vi "Start Shooter Implementation.vi"(8 "Deadband (RPM)":dbl, 10 "Shooter Velocity Setpoint In":dbl, 11 "Shooter":T1) -> (0 "Finished?":bool, 3 "Shooter Velocity Setpoint Out":dbl)   [LabVIEW 2019]
uses:
  <vilib>/Rock Robotics/WPI/MotorControl/WPI_MotorControlDeviceRef.ctl
  <vilib>/Rock Robotics/WPI/MotorControl/WPI_MotorControlType.ctl
  <vilib>/Rock Robotics/SystemInterfaces/DIO/FPGA_DIOPWMChannel.ctl
  <vilib>/Rock Robotics/WPI/PWM/WPI_PWMDeadband.ctl
  <vilib>/Rock Robotics/SystemInterfaces/DIO/FPGA_DIOChannel.ctl
  Turret Published Globals.vi
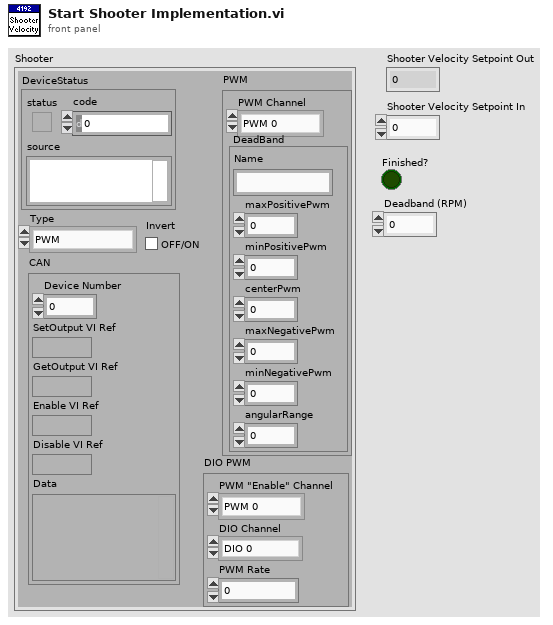
[diagram p1: front panel]
types:
  T1 = typedef "WPI_MotorControlDeviceRef.ctl" = cluster{"DeviceStatus":errorcluster, "Type":T2, "PWM":cluster{"PWM Channel":T3, "DeadBand":T4}, "CAN":cluster{"Device Number":u8, "SetOutput VI Ref":variant, "GetOutput VI Ref":variant, "Enable VI Ref":variant, "Disable VI Ref":variant, "Data":variant}, "Invert":bool, "DIO PWM":cluster{"PWM \"Enable\" Channel":T3, "DIOChannel":T5, "PWM Rate":dbl}}
  T2 = typedef "WPI_MotorControlType.ctl" = enum16{"PWM", "CAN", "DIO PWM"}
  T3 = typedef "FPGA_DIOPWMChannel.ctl" = enum8{"PWM 0", "PWM 1", "PWM 2", "PWM 3", "PWM 4", "PWM 5", "PWM 6", "PWM 7", "PWM 8", "PWM 9", "PWM MXP 0", "PWM MXP 1", "PWM MXP 2", "PWM MXP 3", "PWM MXP 4", "PWM MXP 5", "PWM MXP 6", "PWM MXP 7", "PWM MXP 8", "PWM MXP 9", "Invalid"}
  T4 = typedef "WPI_PWMDeadband.ctl" = cluster{"Name":string, "maxPositivePwm":i32, "minPositivePwm":i32, "centerPwm":i32, "maxNegativePwm":i32, "minNegativePwm":i32, "angularRange":u16}
  T5 = typedef "FPGA_DIOChannel.ctl" = enum8{"DIO 0", "DIO 1", "DIO 2", "DIO 3", "DIO 4", "DIO 5", "DIO 6", "DIO 7", "DIO 8", "DIO 9", "DIO MXP 0", "DIO MXP 1", "DIO MXP 2", "DIO MXP 3", "DIO MXP 4", "DIO MXP 5", "DIO MXP 6", "DIO MXP 7", "DIO MXP 8", "DIO MXP 9", "DIO MXP 10", "DIO MXP 11", "DIO MXP 12", "DIO MXP 13", "DIO MXP 14", "DIO MXP 15", "SPI Port CS1", "SPI Port CS2", "SPI Port CS3", "SPI Port MISO", "SPI Port MOSI", "Invalid"}
  T6 = cluster{"Sensor Velocity":dbl, "Setpoint":dbl, "Applied Output":dbl}
  T7 = cluster{"Shooter Velocity":cluster{"Sensor Velocity":dbl, "Setpoint":dbl, "Applied Output":dbl}, "Turret Position":cluster{"output":dbl, "Horizontal Offset":dbl}, "Hood Position":cluster{"Sensor Velocity":dbl, "Setpoint":dbl, "Applied Output":dbl}, "Shooter PID Constants":cluster{"P Gain":dbl, "I Gain":dbl, "D Gain":dbl, "F Gain":dbl, "I Zone":dbl, "Min Output":dbl, "Max Output":dbl}, "Hood PID Constants":cluster{"P Gain":dbl, "I Gain":dbl, "D Gain":dbl, "F Gain":dbl, "I Zone":dbl, "Min Output":dbl, "Max Output":dbl}, "Turret PID Constants":cluster{"P Gain":dbl, "I Gain":dbl, "D Gain":dbl, "F Gain":dbl, "I Zone":dbl, "Min Output":dbl, "Max Output":dbl}, "Limelight PID Gains":cluster{"proportional gain (Kc)":dbl, "integral time (Ti, min)":dbl, "derivative time (Td, min)":dbl}}
  T8 = cluster{"Shooter Up To Speed?":bool, "Aligned With Target?":bool, "Hood at Angle?":bool, "Shooting?":bool, "Hood Angle":dbl, "Turret Angle":dbl}
  T9 = cluster{"P Gain":dbl, "I Gain":dbl, "D Gain":dbl, "F Gain":dbl, "I Zone":dbl, "Min Output":dbl, "Max Output":dbl}
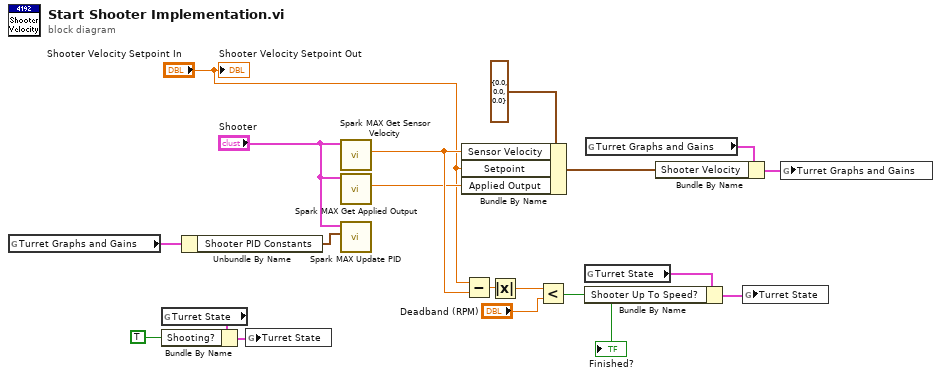
[diagram p0: block diagram]
diagram:
  n1 = global read "Turret Published Globals.vi" "Turret Graphs and Gains"() -> (w11:T7)
  n2 = global read "Turret Published Globals.vi" "Turret State"() -> (w14:T8)
  n3 = Bundle By Name(cluster=w14, "Shooting?"=TRUE) -> (w13:T8)
  n4 = Unbundle By Name(w11) -> ("Shooter PID Constants"=w10:T9)
  n5 = global write "Turret Published Globals.vi" "Turret State"(w13) -> ()
  n6 = call <vilib>:"Spark MAX Get Sensor Velocity.vi"("MotorControlDevRef in"="Shooter") -> ("Sensor Velocity"=w17:dbl)  [unwired: 7 in, 3 out]
  n7 = call <vilib>:"Spark MAX Get Applied Output.vi"("MotorControlDevRef in"="Shooter") -> ("Applied Output"=w16:dbl)  [unwired: 7 in, 3 out]
  n8 = call "Spark MAX Update PID.vi"("MotorControlDeviceRef"="Shooter", "PID Constants"=w10) -> ()  [unwired: 8 in]
  n9 = Bundle By Name(cluster=T6 {"Sensor Velocity"=0.0, "Setpoint"=0.0, "Applied Output"=0.0} ("Shooter Velocity"), "Sensor Velocity"=w17, "Setpoint"="Shooter Velocity Setpoint In", "Applied Output"=w16) -> (w7:T6)
  n10 = Subtract(x="Shooter Velocity Setpoint In", y=w17) -> (x-y=w18:dbl)
  n11 = Absolute Value(x=w18) -> (abs(x)=w19:dbl)
  n12 = Less?(x=w19, y="Deadband (RPM)") -> (x < y?=w3:bool)
  "Finished?" <- w3
  n13 = global read "Turret Published Globals.vi" "Turret State"() -> (w4:T8)
  n14 = Bundle By Name(cluster=w4, "Shooter Up To Speed?"=w3) -> (w5:T8)
  n15 = global read "Turret Published Globals.vi" "Turret Graphs and Gains"() -> (w8:T7)
  n16 = Bundle By Name(cluster=w8, "Shooter Velocity"=w7) -> (w9:T7)
  n17 = global write "Turret Published Globals.vi" "Turret State"(w5) -> ()
  n18 = global write "Turret Published Globals.vi" "Turret Graphs and Gains"(w9) -> ()
  "Shooter Velocity Setpoint Out" <- "Shooter Velocity Setpoint In"
